vi "AIT 1553- Action On Download.vi"(5 "System Definition Dir":path, 6 "IP address":string, 7 "Details Ref":refnum<vi>, 8 "error in (no error)":errorcluster, 10 "ftp session":T2, 11 "Device Item Ref in":T1 format="%.0x") -> (0 "error out":errorcluster, 2 "ftp session out":T2, 3 "Device Item Ref out":T1 format="%.0x")   [LabVIEW 2013, in "AIT 1553 Custom Device.lvlib"]
uses:
  AIT 1553 Custom Device.lvlib
  <vilib>/FTP/ftp0.llb/FTP Session.ctl
  <vilib>/NI Veristand/Custom Device API/Custom Device Item Ref.ctl
  <vilib>/NI Veristand/Custom Device API/Custom Device API.lvlib
  <vilib>/FTP/NI_FTP.lvlib
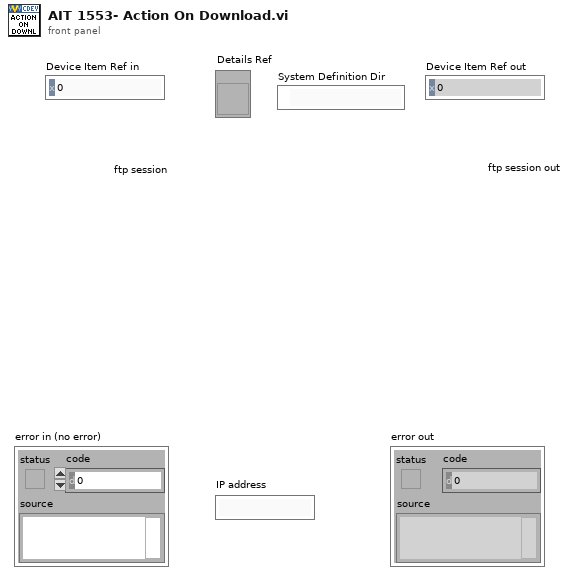
[diagram p1: front panel]
types:
  T1 = typedef "Custom Device API.lvlib/Custom Device Item Ref.ctl" = u64
  T2 = typedef "NI_FTP.lvlib/FTP Session.ctl" = refnum<k5>
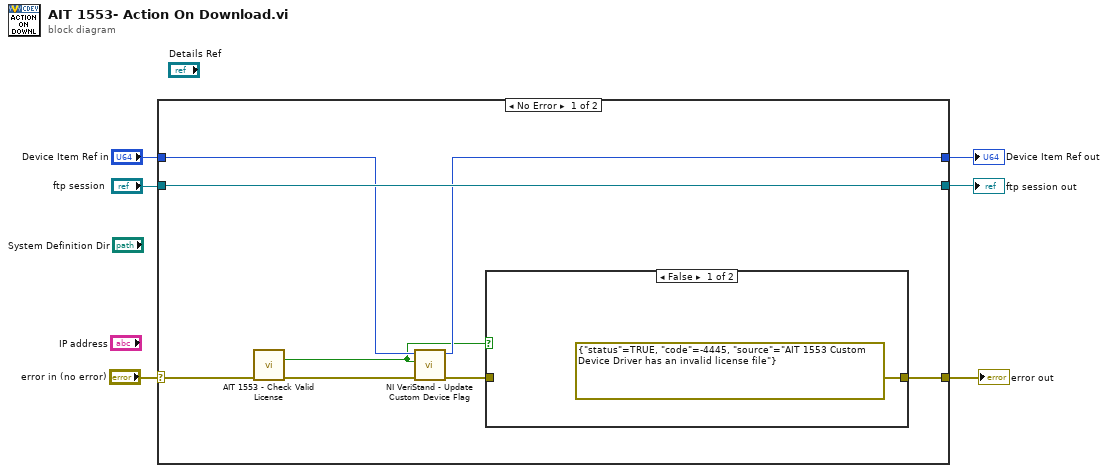
[diagram p0: block diagram]
diagram:
  n1 = case shown="No Error" "error in (no error)" {
    selector: "error in (no error)" -> [w9 w19]
    tunnel: [w10 w19] -> w5
    tunnel: "ftp session" -> [w14 w18]
    tunnel: [w14 w18] -> w3
    tunnel: "Device Item Ref in" -> [w13 w17]
    tunnel: [w12 w17] -> w1
    frame No Error {
      n2 = call "AIT 1553 - Check Valid License.vi"("error in (no error)"=w9) -> ("activated?"=w8:bool, "error out"=w7:errorcluster)  [unwired: 12 in, 1 out]
      n3 = call <vilib>:"NI VeriStand - Update Custom Device Flag.vi"("error in (no error)"=w7, "Is Custom Device Active?"=w8, "Device Ref in"=w13) -> ("error out"=w11:errorcluster, "Device Ref out"=w12:T1)  [unwired: 7 in]
      n4 = case shown="False" w8 {
        tunnel: w11 -> [_ w16]
        tunnel: [errorcluster {"status"=TRUE, "code"=-4445, "source"="AIT 1553 Custom Device Driver has an invalid license file"} ("error out") w16] -> w10
        frame False {
        }
        frame True {
        }
      }
    }
    frame Error {
    }
  }
  "error out" <- w5
  "ftp session out" <- w3
  "Device Item Ref out" <- w1
